vi "SetDO.vi"(6 "value":bool, 8 "error in (no error)":errorcluster caption="错误输入（无错误）", 9 "选择":string(combo), 10 "new reference IN":refnum<k24>, 11 "semaphore IN":T1 caption="信号量输出") -> (0 "error IO":errorcluster, 3 "G_SetDO_1":bool)   [LabVIEW 2017]
uses:
  ADAM-4050DLL.dll
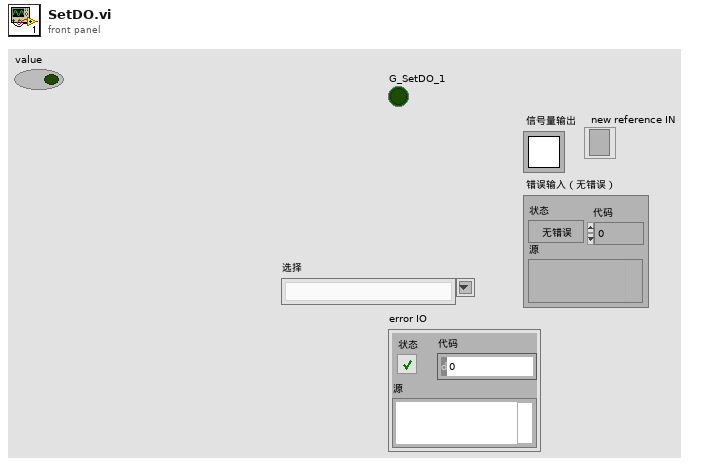
[diagram p1: front panel]
types:
  T1 = typedef "Semaphore RefNum" = refnum<k1>
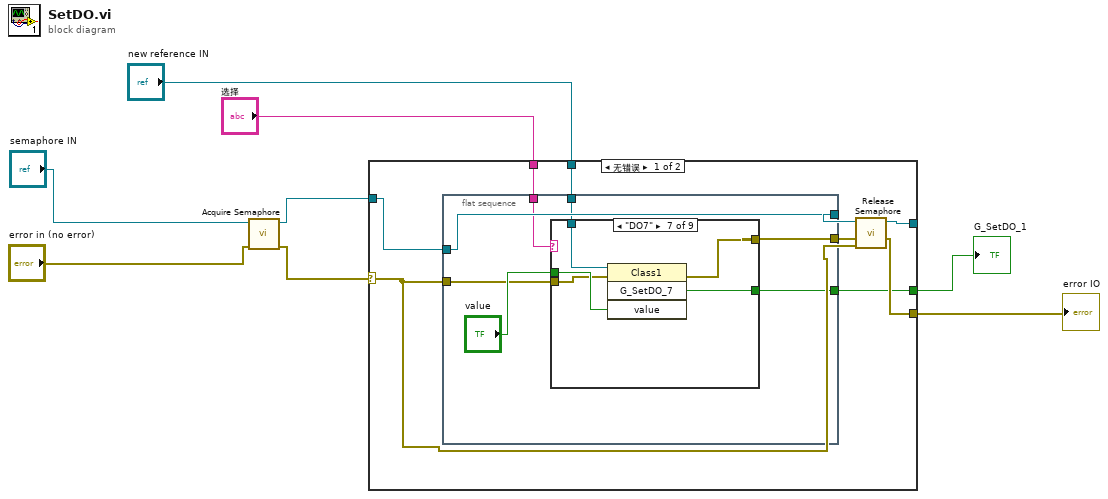
[diagram p0: block diagram]
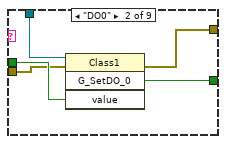
[diagram p3: hidden frame]
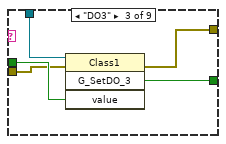
[diagram p4: hidden frame]
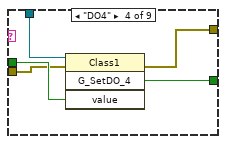
[diagram p5: hidden frame]
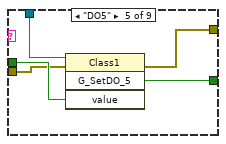
[diagram p6: hidden frame]
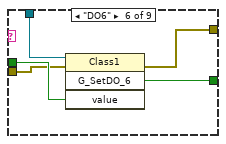
[diagram p7: hidden frame]
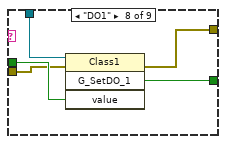
[diagram p8: hidden frame]
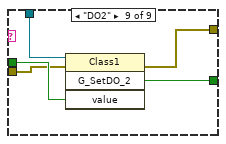
[diagram p9: hidden frame]
diagram:
  n1 = call <vilib>:"Acquire Semaphore.vi"("error in (no error)"="error in (no error)", "semaphore"="semaphore IN") -> ("error out"=w8:errorcluster, "semaphore out"=w7:T1)  [unwired: 3 in, 1 out]
  n2 = case shown="无错误" w8 {
    selector: w8 -> [w11 w65]
    tunnel: w7 -> [w15 w64]
    tunnel: [w13 w64] -> _
    tunnel: [w14 w65] -> w1
    tunnel: "new reference IN" -> [w12 _]
    tunnel: "选择" -> [w10 _]
    tunnel: [w9 _] -> w2
    frame No Error {
      n3 = flat-sequence {
        tunnel: w15 -> [w23]
        tunnel: [w23] -> w16
        tunnel: [w22] -> w14
        tunnel: w12 -> [w20]
        tunnel: w11 -> [w19]
        tunnel: w10 -> [w18]
        tunnel: [w17] -> w9
        frame #0 {
          n4 = case shown="\"DO7\"" w18 {
            tunnel: [_ w28 w33 w38 w43 w48 w53 w58 w63] -> w22
            tunnel: "value" -> [_ w27 w32 w37 w42 w47 w52 w57 w62]
            tunnel: w20 -> [_ w26 w31 w36 w41 w46 w51 w56 w61]
            tunnel: w19 -> [_ w25 w30 w35 w40 w45 w50 w55 w60]
            tunnel: [_ w24 w29 w34 w39 w44 w49 w54 w59] -> w17
            frame "假", Default {
            }
            frame "DO0" {
              n5 = invoke class="Class1" method="G_SetDO_0"(reference=w26, error in=w25, "value"=w27) -> (error out=w28:errorcluster, "G_SetDO_0"=w24:bool)  [unwired: 1 in, 2 out]
            }
            frame "DO3" {
              n6 = invoke class="Class1" method="G_SetDO_3"(reference=w31, error in=w30, "value"=w32) -> (error out=w33:errorcluster, "G_SetDO_3"=w29:bool)  [unwired: 1 in, 2 out]
            }
            frame "DO4" {
              n7 = invoke class="Class1" method="G_SetDO_4"(reference=w36, error in=w35, "value"=w37) -> (error out=w38:errorcluster, "G_SetDO_4"=w34:bool)  [unwired: 1 in, 2 out]
            }
            frame "DO5" {
              n8 = invoke class="Class1" method="G_SetDO_5"(reference=w41, error in=w40, "value"=w42) -> (error out=w43:errorcluster, "G_SetDO_5"=w39:bool)  [unwired: 1 in, 2 out]
            }
            frame "DO6" {
              n9 = invoke class="Class1" method="G_SetDO_6"(reference=w46, error in=w45, "value"=w47) -> (error out=w48:errorcluster, "G_SetDO_6"=w44:bool)  [unwired: 1 in, 2 out]
            }
            frame "DO7" {
              n10 = invoke class="Class1" method="G_SetDO_7"(reference=w51, error in=w50, "value"=w52) -> (error out=w53:errorcluster, "G_SetDO_7"=w49:bool)  [unwired: 1 in, 2 out]
            }
            frame "DO1" {
              n11 = invoke class="Class1" method="G_SetDO_1"(reference=w56, error in=w55, "value"=w57) -> (error out=w58:errorcluster, "G_SetDO_1"=w54:bool)  [unwired: 1 in, 2 out]
            }
            frame "DO2" {
              n12 = invoke class="Class1" method="G_SetDO_2"(reference=w61, error in=w60, "value"=w62) -> (error out=w63:errorcluster, "G_SetDO_2"=w59:bool)  [unwired: 1 in, 2 out]
            }
          }
        }
      }
      n13 = call <vilib>:"Release Semaphore.vi"("error in (no error)"=w11, "semaphore"=w16) -> ("semaphore out"=w13:T1)  [unwired: 4 in, 1 out]
    }
    frame Error {
    }
  }
  "G_SetDO_1" <- w2
  "error IO" <- w1
